vi "FindRobotByID.vi"(8 "error in (no error)":errorcluster, 9 "id":i32, 10 "RobotRef":refnum<class "Robot.lvclass">[](array[class]), 11 "Utilities in":refnum<class "Utilities.lvclass">) -> (0 "error out":errorcluster, 1 "index":i32, 2 "Robot":refnum<class "Robot.lvclass">, 3 "Utilities out":refnum<class "Utilities.lvclass">)   [LabVIEW 2018, in "Utilities.lvclass"]
uses:
  Utilities.lvclass
  Robot_class/Robot.lvclass
  Robot_class/Robot.lvclass/Robot.ctl
  Robot_class/Read id.vi
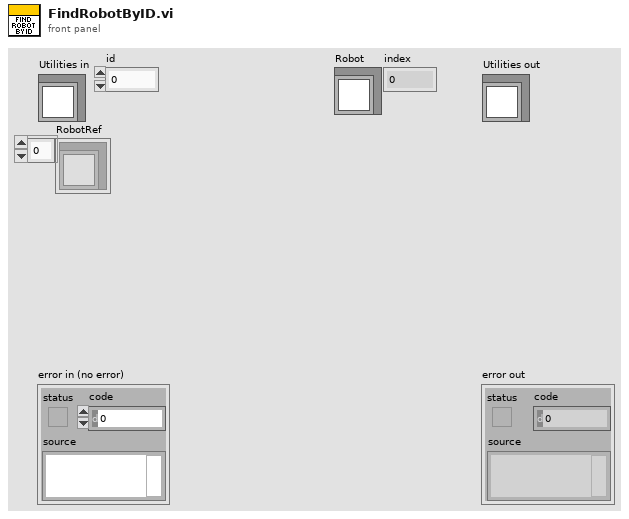
[diagram p1: front panel]
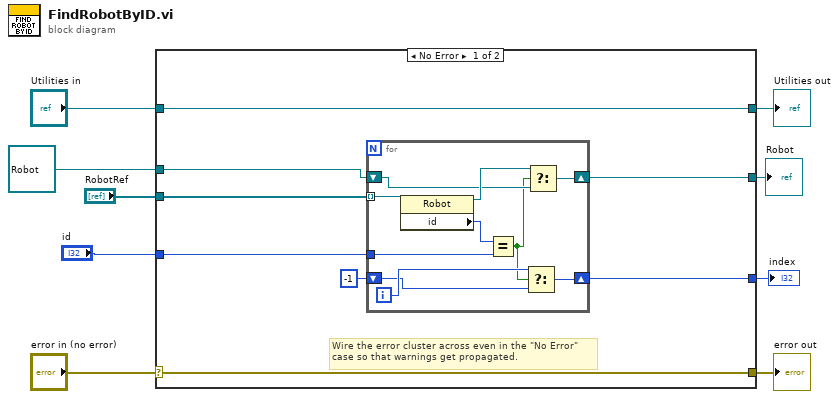
[diagram p0: block diagram]
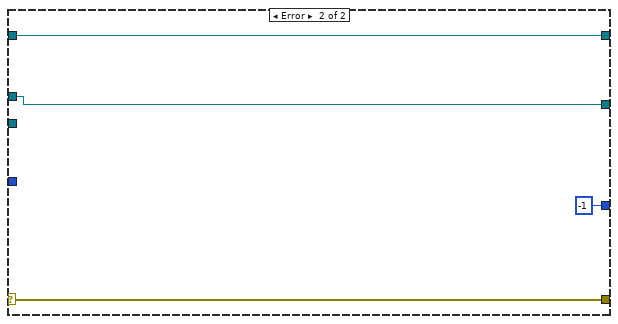
[diagram p2: hidden frame]
diagram:
  n1 = case shown="No Error" "error in (no error)" {
    selector: "error in (no error)" -> [w16 w31]
    tunnel: [w16 w31] -> w8
    tunnel: [w17 w30] -> w6
    tunnel: "Utilities in" -> [w17 w30]
    tunnel: "RobotRef" -> [w15 _]
    tunnel: "id" -> [w14 _]
    tunnel: [w13 w29] -> w3
    tunnel: refnum<class "Robot.lvclass"> refnum ("Robot") -> [w12 w29]
    tunnel: [w10 -1] -> w1
    frame No Error {
      # "Wire the error cluster across even in the \"No Error\"\ncase so that warnings get propagated."
      n2 = for {
        tunnel: w15 -> [w27] mode=indexing
        tunnel: w14 -> [w25]
        shift-right: [w23] -> w13
        shift-left: w12 -> [w22]
        shift-right: [w19] -> w10
        shift-left: -1 -> [w18]
        i -> [w21]
        n3 = property class="Robot"(reference=w27) -> (reference out=w24:refnum<class "Robot.lvclass">, "id"=w26:i32)  [unwired: 1 in, 1 out]
        n4 = Equal?(x=w26, y=w25) -> (x = y?=w20:bool)
        n5 = Select(t=w21, s=w20, f=w18) -> (s? t:f=w19:i32)
        n6 = Select(t=w24, s=w20, f=w22) -> (s? t:f=w23:refnum<class "Robot.lvclass">)
      }
    }
    frame Error {
    }
  }
  "error out" <- w8
  "Utilities out" <- w6
  "Robot" <- w3
  "index" <- w1
